vi "Render.vi"(8 "error in":errorcluster, 10 "Renderer in":refnum<class "Renderer.lvclass">, 11 "TAF Proj Document Type:FrontPanelGUI in":refnum<class "FrontPanelGUI.lvclass">) -> (0 "error out":errorcluster, 3 "Sections out":refnum<class "Section.lvclass">[](array[class]))   [LabVIEW 2021, in "TAF Proj Document Type.lvlib" / "FrontPanelGUI.lvclass"]
uses:
  <vilib>/Wovalab/AntiDoc/Document Type/Add-ons/LabVIEW TAF Project/FrontPanelGUI/FrontPanelGUI.lvclass
  C:/Program Files (x86)/National Instruments/LabVIEW 2021/vi.lib/Wovalab/AntiDoc/Bloc/Bloc.lvclass
  <vilib>/Wovalab/AntiDoc/Renderer/Renderer.lvclass
  <vilib>/Wovalab/AsciiDoc for LabVIEW/Section/Section.lvclass
  <vilib>/Wovalab/AntiDoc/Renderer/Renderer.lvclass/Renderer.ctl
  <vilib>/Wovalab/AntiDoc/Bloc/Bloc.lvclass/Bloc.ctl
  <vilib>/Wovalab/AsciiDoc for LabVIEW/Table/Table Attributes--cluster.ctl
  <vilib>/Wovalab/AsciiDoc for LabVIEW/Table/Frame--enum.ctl
  <vilib>/Wovalab/AsciiDoc for LabVIEW/Table/Grid--enum.ctl
  <vilib>/Wovalab/AsciiDoc for LabVIEW/Table/Stripes--enum.ctl
  <vilib>/Wovalab/AsciiDoc for LabVIEW/Table/Column Attributes--cluster.ctl
  <vilib>/Wovalab/AsciiDoc for LabVIEW/Table/Horizontal Alignment--enum.ctl
  <vilib>/Wovalab/AsciiDoc for LabVIEW/Table/Vertical Alignment--enum.ctl
  <vilib>/Wovalab/AsciiDoc for LabVIEW/Table/Style--enum.ctl
  <vilib>/Wovalab/AsciiDoc for LabVIEW/Table/Table.lvclass/Table.ctl
  <vilib>/Wovalab/AntiDoc/Renderer/Read Image Folder Path.vi
  <vilib>/Wovalab/AntiDoc/Bloc/Read Name.vi
  <vilib>/Wovalab/AsciiDoc for LabVIEW/Table/Table.lvclass
  C:/Program Files (x86)/National Instruments/LabVIEW 2021/vi.lib/Wovalab/AsciiDoc for LabVIEW/Adoc-Bloc/Bloc.lvclass
  <vilib>/Wovalab/AsciiDoc for LabVIEW/Section/Add Bloc (array).vi
  <vilib>/Wovalab/AntiDoc/Utilities/Utilities.lvlib
  <vilib>/Wovalab/AntiDoc/Document Type/Add-ons/LabVIEW TAF Project/Vi/Vi.lvclass
  C:/Program Files (x86)/National Instruments/LabVIEW 2021/vi.lib/Wovalab/AsciiDoc for LabVIEW/Table/Table.lvclass
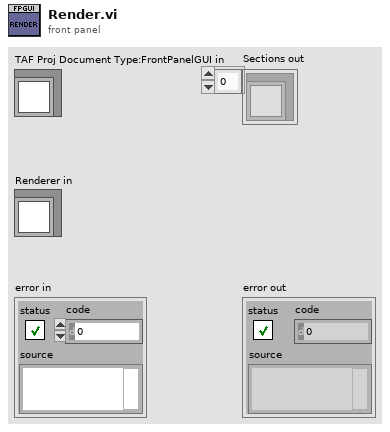
[diagram p1: front panel]
types:
  T1 = typedef "imagedata.ctl" = cluster{"image type":i32, "image depth":i32, "image":u8[], "mask":u8[], "colors":u32[], "Rectangle":cluster{"left":i16, "top":i16, "right":i16, "bottom":i16}}
  T2 = cluster{"VI Name":string, "Lib Name":string, "Controls":string[], "ControlImage":T1[], "Descriptions":string[]}[]
  T3 = typedef "Wovalab_lib_AsciiDoctor.lvlib/Table.lvclass/Column Attributes--cluster.ctl" = cluster{"Width":u16, "Horizontal Alignment":T4, "Vertical Alignment":T5, "Style":T6}
  T4 = typedef "Wovalab_lib_AsciiDoctor.lvlib/Table.lvclass/Horizontal Alignment--enum.ctl" = enum16{"Left", "Center", "Right"}
  T5 = typedef "Wovalab_lib_AsciiDoctor.lvlib/Table.lvclass/Vertical Alignment--enum.ctl" = enum16{"Top", "Middle", "Bottom"}
  T6 = typedef "Wovalab_lib_AsciiDoctor.lvlib/Table.lvclass/Style--enum.ctl" = enum16{"None", "AsciiDoc", "Emphasis", "Header", "Literal", "Monospaced", "Strong", "Verse"}
  T7 = typedef "Wovalab_lib_AsciiDoctor.lvlib/Table.lvclass/Table Attributes--cluster.ctl" = cluster{"autowidth":bool, "Witdth":u8, "Frame":T8, "Grid":T9, "Stripes":T10}
  T8 = typedef "Wovalab_lib_AsciiDoctor.lvlib/Table.lvclass/Frame--enum.ctl" = enum16{"all", "topbot", "sides", "none"}
  T9 = typedef "Wovalab_lib_AsciiDoctor.lvlib/Table.lvclass/Grid--enum.ctl" = enum16{"all", "rows", "cols", "none"}
  T10 = typedef "Wovalab_lib_AsciiDoctor.lvlib/Table.lvclass/Stripes--enum.ctl" = enum16{"none", "even", "odd", "all", "hover"}
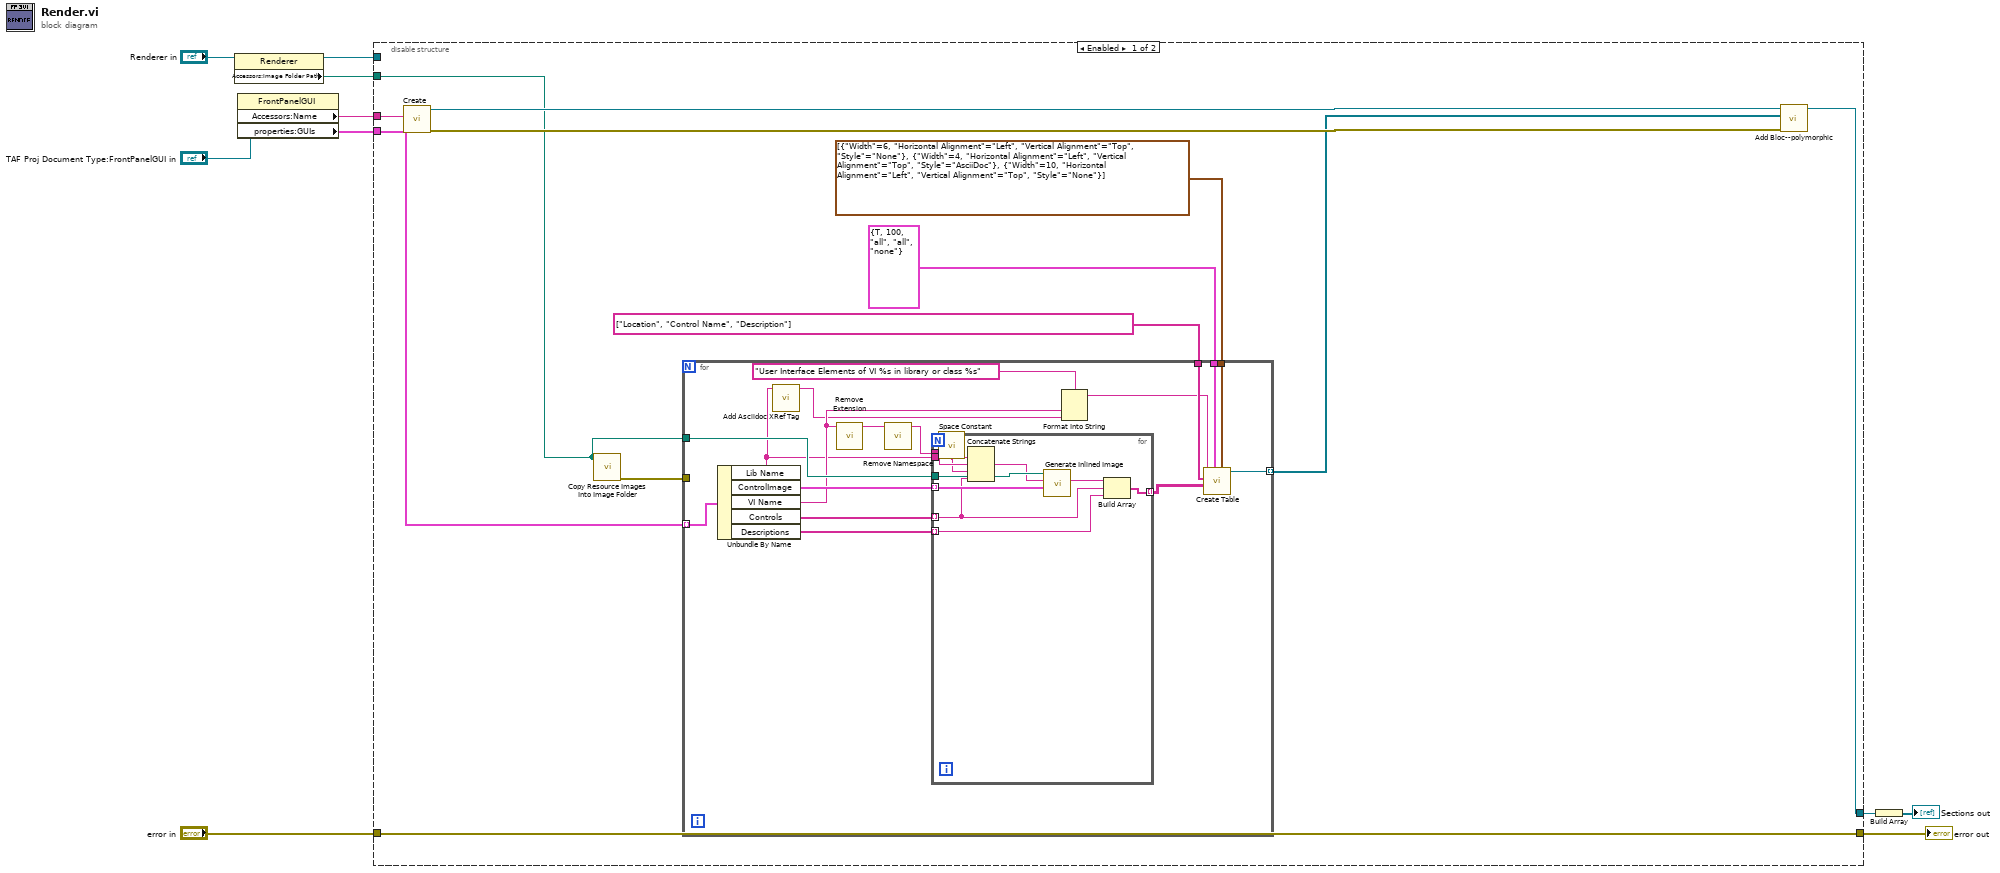
[diagram p0: block diagram]
diagram:
  n1 = property class="Renderer"(reference="Renderer in") -> (reference out=w3:refnum<class "Renderer.lvclass">, "Accessors:Image Folder Path"=w2:path)  [unwired: 1 in, 1 out]
  n2 = property class="FrontPanelGUI"(reference="TAF Proj Document Type:FrontPanelGUI in") -> ("Accessors:Name"=w6:string, "properties:GUIs"=w1:T2)  [unwired: 1 in, 2 out]
  n3 = disable-structure shown="Enabled" {
    disable-tunnel: "error in" -> [w12 _]
    disable-tunnel: [w12 _] -> w9
    disable-tunnel: w3 -> [_ _]
    disable-tunnel: w6 -> [w20 _]
    disable-tunnel: [w13 _] -> w5
    disable-tunnel: w2 -> [w19 _]
    disable-tunnel: w1 -> [w18 _]
    frame Enabled {
      n4 = call <vilib>:"Create.vi"("Title"=w20) -> ("error out"=w22:errorcluster, "Section out"=w21:refnum<class "Section.lvclass">)  [unwired: 9 in]
      n5 = call <vilib>:"Copy Resource Images Into Image Folder.vi"("Image Folder Path"=w19) -> ("error out"=w11:errorcluster)  [unwired: 9 in, 1 out]
      n6 = for {
        tunnel: w18 -> [w39] mode=indexing
        tunnel: w19 -> [w35]
        tunnel: T3[] [{"Width"=6, "Horizontal Alignment"=enum."Left", "Vertical Alignment"=enum."Top", "Style"=enum."None"}, {"Width"=4, "Horizontal Alignment"=enum."Left", "Vertical Alignment"=enum."Top", "Style"=enum."AsciiDoc"}, {"Width"=10, "Horizontal Alignment"=enum."Left", "Vertical Alignment"=enum."Top", "Style"=enum."None"}] ("Column Attributes") -> [w32]
        tunnel: T7 {"autowidth"=TRUE, "Witdth"=100, "Frame"=enum."all", "Grid"=enum."all", "Stripes"=enum."none"} ("Table Attributes") -> [w31]
        tunnel: string[] ["Location", "Control Name", "Description"] ("Header") -> [w30]
        tunnel: [w29] -> w14 mode=indexing
        tunnel: w11 -> [_]
        n7 = Unbundle By Name(w39) -> ("Lib Name"=w24:string, "ControlImage"=w36:T1[], "VI Name"=w25:string, "Controls"=w37:string[], "Descriptions"=w34:string[])
        n8 = call <vilib>:"Add Asciidoc XRef Tag.vi"("String In"=w24) -> ("String out"=w23:string)  [unwired: 10 in]
        n9 = call <vilib>:"Remove Extension.vi"("File Name"=w25) -> ("File Name Without Extension"=w38:string)  [unwired: 10 in]
        n10 = call <vilib>:"Remove Namespace.vi"("Vi Name"=w38) -> ("Vi Name Without Namespace"=w26:string)  [unwired: 10 in]
        n11 = for {
          tunnel: w37 -> [w40] mode=indexing
          tunnel: w36 -> [w48] mode=indexing
          tunnel: w35 -> [w49]
          tunnel: w34 -> [w46] mode=indexing
          tunnel: [w45] -> w27 mode=indexing
          tunnel: w26 -> [w43]
          tunnel: w24 -> [w44]
          n12 = call <vilib>:"Space Constant.vi"() -> ("String"=w41:string)
          n13 = Concatenate Strings(w44, w41, w43, w41, w40) -> (w42:string)
          n14 = call <vilib>:"Generate Inlined Image.vi"("empty"=w48, "Name"=w42, "Image Folder Path"=w49) -> ("Image String"=w47:string)  [unwired: 6 in, 2 out]
          n15 = Build Array(w47, w40, w46) -> (w45:string[])
        }
        n16 = Format Into String(format string="User Interface Elements of VI %s in library or class %s" ("Title"), w25, w23) -> (resulting string=w28:string)  [unwired: 2 in, 1 out]
        n17 = call <vilib>:"Create Table.vi"("Column Attributes"=w32, "Table Attributes"=w31, "Content"=w27, "Header"=w30, "Title"=w28) -> ("Table out"=w29:refnum<class "Table.lvclass">)  [unwired: 5 in, 1 out]
      }
      n18 = call-poly <vilib>:"Add Bloc--polymorphic.vi"("error in"=w22, "Bloc"=w14, "Section in"=w21) -> ("Section out"=w13:refnum<class "Section.lvclass">)  [unwired: 7 in, 1 out]
    }
    frame Disabled {
    }
  }
  "error out" <- w9
  n19 = Build Array(w5) -> (→"Sections out":refnum<class "Section.lvclass">[])
